vi "ClassAndMethodVIDescriptionEditor.vi"() -> ()   [LabVIEW 2021]
panel:
  in  "Refresh":bool
  in  "Folder Search":string
  in  "Childeren":bool
  in  "Tree":string(tree)
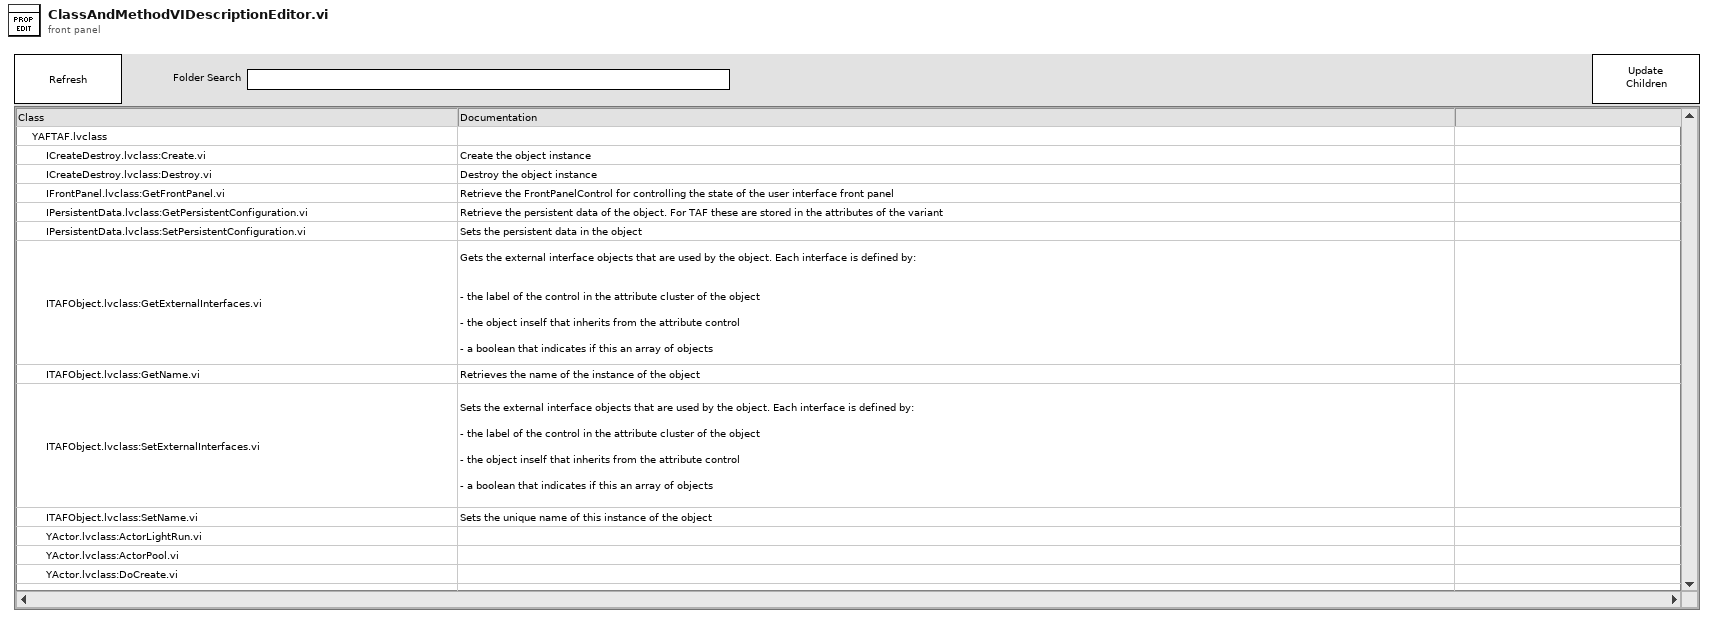
[diagram p1: front panel]
types:
  T1 = enum32{"invalid scope", "public", "private", "protected", "community"}
  T2 = cluster{"Left Cell String":string, "Child Text":string[], "Child Tag":string, "Item Indent":i32, "Child Only?":bool, "Glyph Index":i32}
  T3 = cluster{"Project.ActiveProject":refnum<vi>, "My Computer":refnum<vi>, "All Descendents":refnum<vi>[], "All Descendents":refnum<vi>[], refnum<vi>[]}
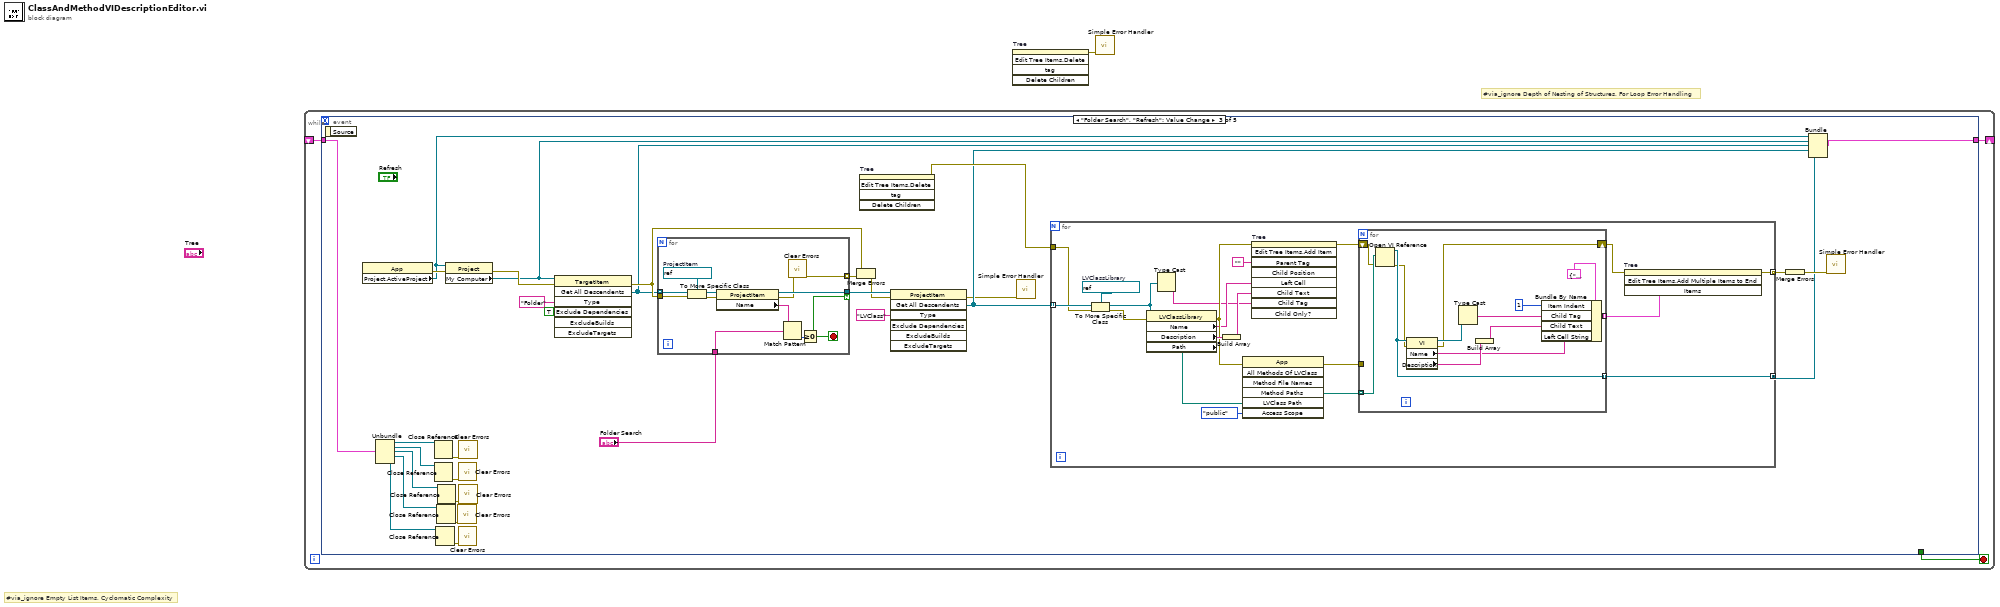
[diagram p0: block diagram]
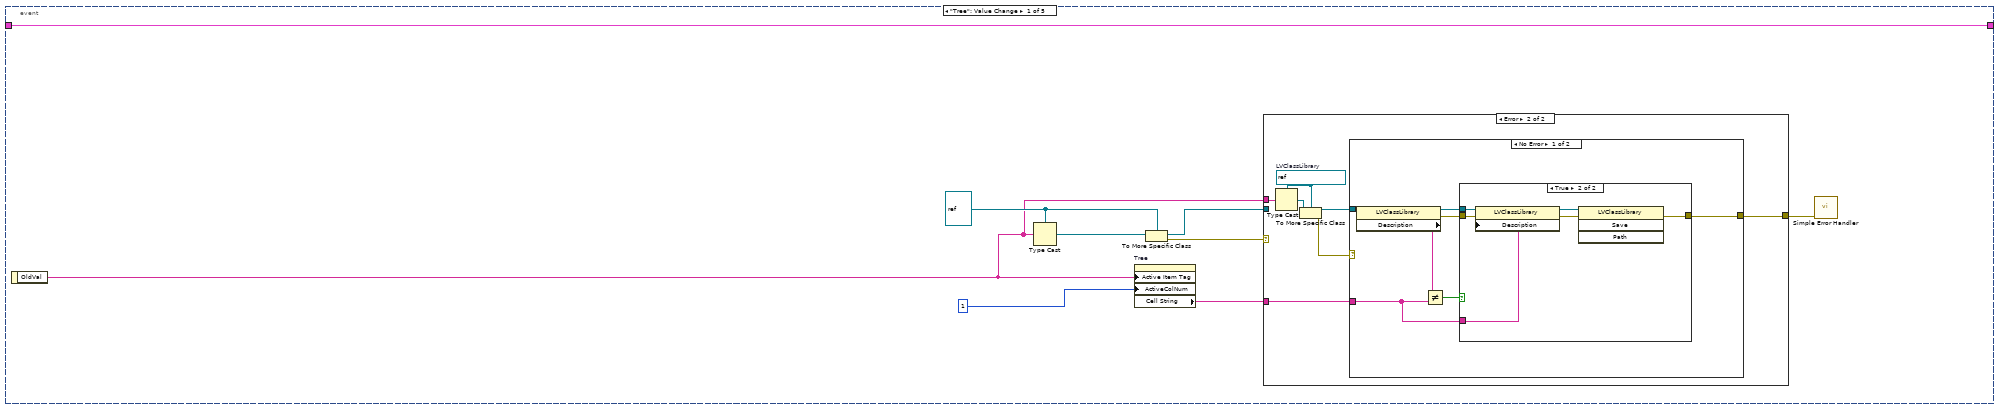
[diagram p2: hidden frame]
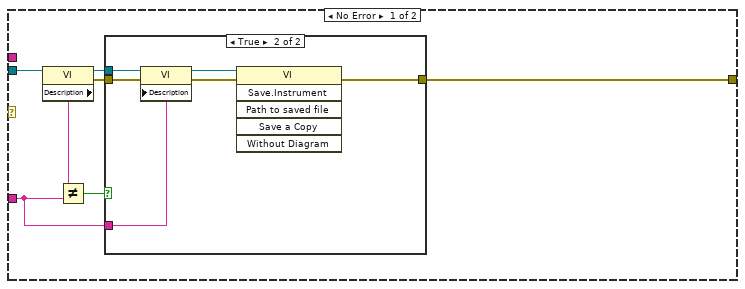
[diagram p3: hidden frame]
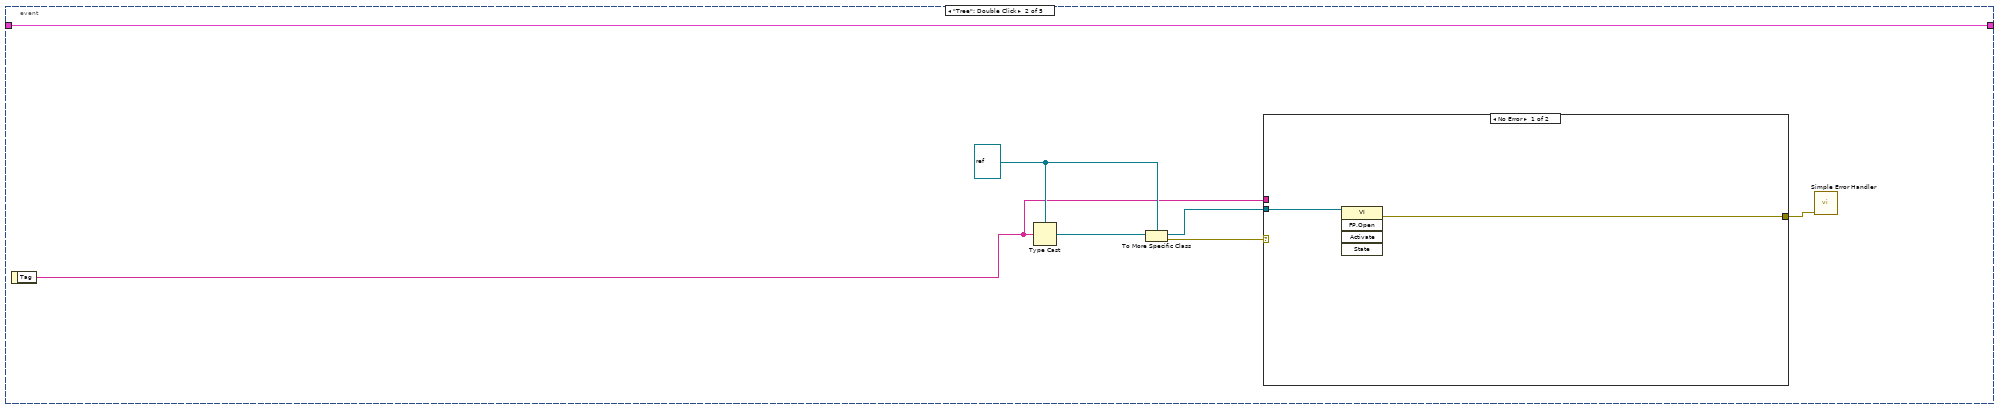
[diagram p7: hidden frame]
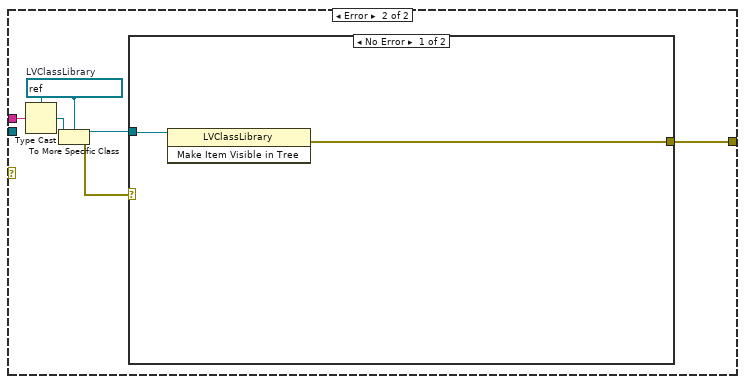
[diagram p8: hidden frame]
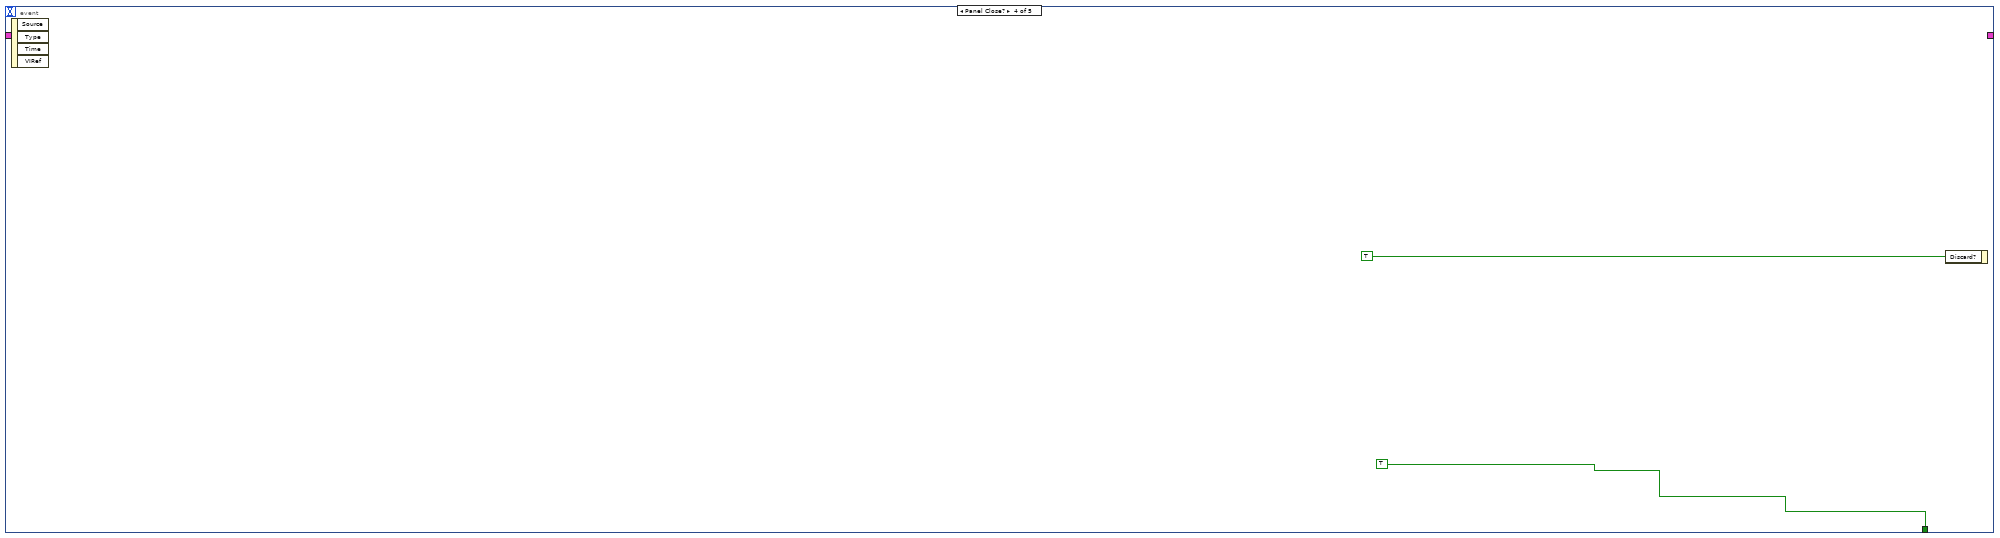
[diagram p10: hidden frame]
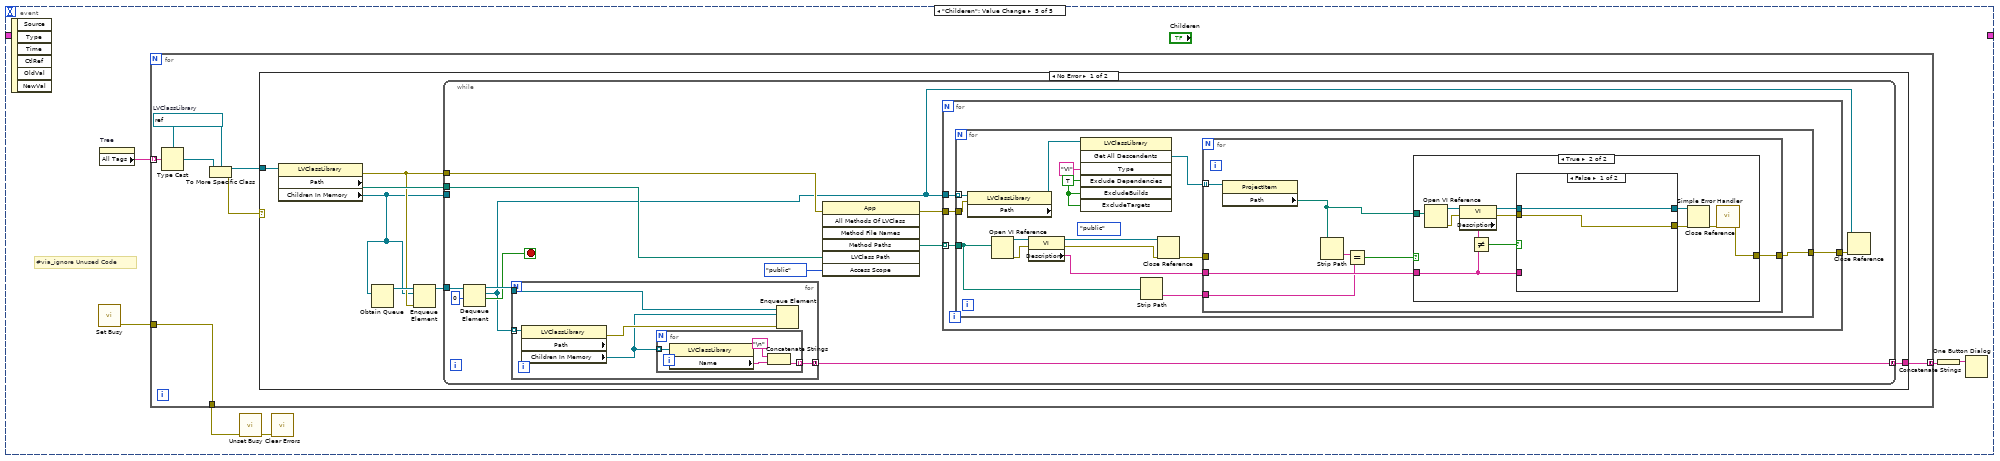
[diagram p11: hidden frame]
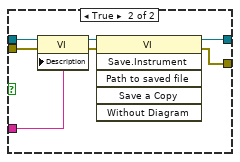
[diagram p13: hidden frame]
diagram:
  # "#via_ignore Depth of Nesting of Structures, For Loop Error Handling"
  # "#via_ignore Empty List Items, Cyclomatic Complexity"
  n1 = while {
    shift-right: [w4] -> _
    shift-left: _ -> [w3]
    stop <- w2 stop-if-true
    n2 = event shown="[2] \"Folder Search\", \"Refresh\": Value Change" {
      selector: _ -> [_ _ _ _ _]
      dyn-events: _ -> [_ _ _ _ _]
      timeout: _ -> [_ _ _ _ _]
      tunnel: [w8 w52 w81 _ _] -> w4
      tunnel: w3 -> [w8 w52 w80 _ _]
      tunnel: [_ _ _ TRUE _] -> w2
      event "Tree": Value Change {
        w12 = refnum<vi> refnum ("reference out")
        n3 = event-data() -> ("OldVal"=w6:string)  [unwired: 1 in]
        n4 = Type Cast(type=w12, x=w6) -> (*(type *) &x=w7:refnum<vi>)
        n5 = property on="Tree" class="Tree (strict)"("Active Item Tag"=w6, "ActiveColNum"=1 ("Active Cell:Active Column Number")) -> ("Cell String"=w9:string)  [unwired: 2 in, 2 out]
        n6 = To More Specific Class(target class=w12, reference=w7) -> (specific class reference=w10:refnum<vi>, error out=w11:errorcluster)  [unwired: 1 in]
        n7 = case shown="Error" w11 {
          tunnel: w10 -> [w20 _]
          tunnel: w9 -> [w16 w34]
          tunnel: w6 -> [_ w31]
          tunnel: [w14 w28] -> w5
          frame No Error {
            n8 = property class="VI"(reference=w20) -> (reference out=w17:refnum<vi>, error out=w15:errorcluster, "Description"=w19:string)  [unwired: 1 in]
            n9 = Not Equal?(x=w19, y=w16) -> (x != y?=w18:bool)
            n10 = case shown="True" w18 {
              tunnel: w17 -> [_ w27]
              tunnel: w16 -> [_ w26]
              tunnel: w15 -> [w21 w23]
              tunnel: [w21 w22] -> w14
              frame False {
              }
              frame True {
                n11 = property class="VI"(reference=w27, error in=w23, "Description"=w26) -> (reference out=w25:refnum<vi>, error out=w24:errorcluster)
                n12 = invoke class="VI" method="Save.Instrument"(reference=w25, error in=w24) -> (error out=w22:errorcluster)  [unwired: 4 in, 5 out]
              }
            }
          }
          frame Error {
            w29 = refnum<vi> refnum  # LVClassLibrary
            n13 = Type Cast(type=w29, x=w31) -> (*(type *) &x=w30:refnum<vi>)
            n14 = To More Specific Class(target class=w29, reference=w30) -> (specific class reference=w33:refnum<vi>, error out=w32:errorcluster)  [unwired: 1 in]
            n15 = case shown="No Error" w32 {
              tunnel: w34 -> [w38 _]
              tunnel: w33 -> [w36 _]
              tunnel: [w35 _] -> w28
              frame No Error {
                n16 = property class="LVClassLibrary"(reference=w36) -> (reference out=w39:refnum<vi>, error out=w37:errorcluster, "Description"=w41:string)  [unwired: 1 in]
                n17 = Not Equal?(x=w41, y=w38) -> (x != y?=w40:bool)
                n18 = case shown="True" w40 {
                  tunnel: w39 -> [_ w48]
                  tunnel: w38 -> [_ w47]
                  tunnel: w37 -> [w42 w44]
                  tunnel: [w42 w43] -> w35
                  frame False {
                  }
                  frame True {
                    n19 = property class="LVClassLibrary"(reference=w48, error in=w44, "Description"=w47) -> (reference out=w46:refnum<vi>, error out=w45:errorcluster)
                    n20 = invoke class="LVClassLibrary" method="Save"(reference=w46, error in=w45) -> (error out=w43:errorcluster)  [unwired: 2 in, 3 out]
                  }
                }
              }
              frame Error {
              }
            }
          }
        }
        n21 = call <vilib>:"Simple Error Handler.vi"("error in (no error)"=w5) -> ()  [unwired: 4 in, 5 out]
      }
      event "Tree": Double Click {
        w55 = refnum<vi> refnum ("reference out")
        n22 = event-data() -> ("Tag"=w50:string)  [unwired: 1 in]
        n23 = Type Cast(type=w55, x=w50) -> (*(type *) &x=w51:refnum<vi>)
        n24 = To More Specific Class(target class=w55, reference=w51) -> (specific class reference=w53:refnum<vi>, error out=w54:errorcluster)  [unwired: 1 in]
        n25 = case shown="No Error" w54 {
          tunnel: w53 -> [w57 _]
          tunnel: w50 -> [_ w61]
          tunnel: [w56 w58] -> w49
          frame No Error {
            n26 = invoke class="VI" method="FP.Open"(reference=w57) -> (error out=w56:errorcluster)  [unwired: 4 in, 4 out]
          }
          frame Error {
            w59 = refnum<vi> refnum  # LVClassLibrary
            n27 = Type Cast(type=w59, x=w61) -> (*(type *) &x=w60:refnum<vi>)
            n28 = To More Specific Class(target class=w59, reference=w60) -> (specific class reference=w63:refnum<vi>, error out=w62:errorcluster)  [unwired: 1 in]
            n29 = case shown="No Error" w62 {
              tunnel: w63 -> [w65 _]
              tunnel: [w64 _] -> w58
              frame No Error {
                n30 = invoke class="LVClassLibrary" method="Make Item Visible in Tree"(reference=w65) -> (error out=w64:errorcluster)  [unwired: 2 in, 2 out]
              }
              frame Error {
              }
            }
          }
        }
        n31 = call <vilib>:"Simple Error Handler.vi"("error in (no error)"=w49) -> ()  [unwired: 4 in, 5 out]
      }
      event "Folder Search", "Refresh": Value Change {
        w88 = TRUE ("ExcludeDependencies")
        n32 = event-data() -> ()  [unwired: 1 in, 1 out]
        n33 = property class="App"() -> (error out=w93:errorcluster, "Project.ActiveProject"=w85:refnum<vi>)  [unwired: 2 in, 1 out]
        n34 = Unbundle(w80) -> ("Project.ActiveProject"=w79:refnum<vi>, "My Computer"=w78:refnum<vi>, "All Descendents"=w77:refnum<vi>[], "All Descendents"=w76:refnum<vi>[], w69:refnum<vi>[])
        n35 = Close Reference(reference=w79) -> (error out=w75:errorcluster)  [unwired: 1 in]
        n36 = Close Reference(reference=w78) -> (error out=w74:errorcluster)  [unwired: 1 in]
        n37 = Close Reference(reference=w69) -> (error out=w71:errorcluster)  [unwired: 1 in]
        n38 = Close Reference(reference=w76) -> (error out=w72:errorcluster)  [unwired: 1 in]
        n39 = Close Reference(reference=w77) -> (error out=w73:errorcluster)  [unwired: 1 in]
        n40 = property class="Project"(reference=w85, error in=w93) -> (error out=w94:errorcluster, "My Computer"=w84:refnum<vi>)  [unwired: 1 out]
        n41 = call <vilib>:"Clear Errors.vi"("error in (no error)"=w72) -> ()  [unwired: 5 in, 2 out]
        n42 = call <vilib>:"Clear Errors.vi"("error in (no error)"=w74) -> ()  [unwired: 5 in, 2 out]
        n43 = call <vilib>:"Clear Errors.vi"("error in (no error)"=w71) -> ()  [unwired: 5 in, 2 out]
        n44 = call <vilib>:"Clear Errors.vi"("error in (no error)"=w75) -> ()  [unwired: 5 in, 2 out]
        n45 = call <vilib>:"Clear Errors.vi"("error in (no error)"=w73) -> ()  [unwired: 5 in, 2 out]
        n46 = invoke class="TargetItem" method="Get All Descendents"(reference=w84, error in=w94, "Type"="Folder", "Exclude Dependencies"=w88, "ExcludeBuilds"=w88, "ExcludeTargets"=w88) -> (error out=w95:errorcluster, "All Descendents"=w83:refnum<vi>[])  [unwired: 1 in, 5 out]
        n47 = for {
          tunnel: w83 -> [w141] mode=indexing
          tunnel: [w136] -> w91 if=w134
          tunnel: w95 -> [w133]
          tunnel: "Folder Search" -> [w131]
          tunnel: [w130] -> w66 mode=indexing
          stop <- w134 stop-if-true
          w140 = refnum<vi> refnum  # ProjectItem
          n48 = To More Specific Class(target class=w140, reference=w141, error in=w133) -> (specific class reference=w139:refnum<vi>, error out=w138:errorcluster)
          n49 = property class="ProjectItem"(reference=w139, error in=w138) -> (reference out=w136:refnum<vi>, error out=w132:errorcluster, "Name"=w137:string)
          n50 = Match Pattern(string=w137, regular expression=w131) -> (offset past match=w135:i32)  [unwired: 1 in, 3 out]
          n51 = call <vilib>:"Clear Errors.vi"("error in (no error)"=w132) -> ("error out"=w130:errorcluster)  [unwired: 5 in, 1 out]
          n52 = Greater Or Equal To 0?(x=w135) -> (x >= 0?=w134:bool)
        }
        n53 = Merge Errors(w95, w66) -> (w67:errorcluster)
        n54 = invoke on="Tree" class="Tree (strict)" method="Edit Tree Items.Delete"() -> (error out=w92:errorcluster)  [unwired: 5 in, 4 out]
        n55 = invoke class="ProjectItem" method="Get All Descendents"(reference=w91, error in=w67, "Type"="LVClass") -> (error out=w68:errorcluster, "All Descendents"=w82:refnum<vi>[])  [unwired: 4 in, 5 out]
        n56 = call <vilib>:"Simple Error Handler.vi"("error in (no error)"=w68) -> ()  [unwired: 4 in, 5 out]
        n57 = for {
          tunnel: w82 -> [w116] mode=indexing
          tunnel: w92 -> [w101]
          tunnel: [w108] -> w87 mode=indexing
          tunnel: [w104] -> w70 mode=concatenating
          w115 = refnum<vi> refnum  # LVClassLibrary
          n58 = To More Specific Class(target class=w115, reference=w116, error in=w101) -> (specific class reference=w112:refnum<vi>, error out=w111:errorcluster)
          n59 = property class="LVClassLibrary"(reference=w112, error in=w111) -> (error out=w103:errorcluster, "Name"=w98:string, "Description"=w113:string, "Path"=w107:path)  [unwired: 1 out]
          n60 = Type Cast(x=w112) -> (*(type *) &x=w97:string)  [unwired: 1 in]
          n61 = Build Array(w113) -> (w100:string[])
          n62 = invoke class="App" method="All Methods Of LVClass"(error in=w103, "LVClass Path"=w107, "Access Scope"=T1."public") -> (error out=w102:errorcluster, "Method Paths"=w105:path[])  [unwired: 4 in, 5 out]
          n63 = invoke on="Tree" class="Tree (strict)" method="Edit Tree Items.Add Item"(error in=w103, "Parent Tag"="", "Left Cell"=w98, "Child Text"=w100, "Child Tag"=w97) -> (error out=w110:errorcluster)  [unwired: 4 in, 8 out]
          n64 = for {
            tunnel: [w127] -> w114 mode=indexing
            shift-right: [w121] -> w109
            shift-left: w110 -> [w118]
            tunnel: w105 -> [w120] mode=indexing
            tunnel: [w119] -> w104 mode=indexing
            tunnel: w102 -> [_]
            n65 = Open VI Reference(vi path=w120, error in (no error)=w118) -> (vi reference=w119:refnum<vi>, error out=w117:errorcluster)  [unwired: 4 in]
            n66 = property class="VI"(reference=w119, error in=w117) -> (reference out=w122:refnum<vi>, error out=w121:errorcluster, "Name"=w124:string, "Description"=w126:string)
            n67 = Type Cast(x=w122) -> (*(type *) &x=w123:string)  [unwired: 1 in]
            n68 = Build Array(w126) -> (w125:string[])
            n69 = Bundle By Name(cluster=T2 {"Left Cell String"="", "Child Text"=[], "Child Tag"="", "Item Indent"=0, "Child Only?"=FALSE, "Glyph Index"=0} ("Item"), "Item Indent"=1, "Child Tag"=w123, "Child Text"=w125, "Left Cell String"=w124) -> (w127:T2)
          }
          n70 = invoke on="Tree" class="Tree (strict)" method="Edit Tree Items.Add Multiple Items to End"(error in=w109, "Items"=w114) -> (error out=w108:errorcluster)  [unwired: 2 in, 3 out]
        }
        n71 = Merge Errors(w87) -> (w86:errorcluster)
        n72 = Bundle("Project.ActiveProject"=w85, "My Computer"=w84, "All Descendents"=w83, "All Descendents"=w82, w70) -> (w81:T3)  [unwired: 1 in]
        n73 = call <vilib>:"Simple Error Handler.vi"("error in (no error)"=w86) -> ()  [unwired: 4 in, 5 out]
      }
      event Panel Close? {
        n74 = event-data() -> ()  [unwired: 1 in, 4 out]
        n75 = event-data("Discard?"=TRUE) -> ()  [unwired: 1 in, 1 out]
      }
      event "Childeren": Value Change {
        # "#via_ignore Unused Code"
        n76 = event-data() -> ()  [unwired: 1 in, 6 out]
        n77 = call <vilib>:"Set Busy.vi"() -> ("error out"=w148:errorcluster)  [unwired: 10 in, 1 out]
        n78 = property on="Tree" class="Tree (strict)"() -> ("All Tags"=w149:string[])  [unwired: 2 in, 2 out]
        n79 = for {
          tunnel: w149 -> [w152] mode=indexing
          tunnel: [w151] -> w147
          tunnel: w148 -> [w151]
          tunnel: [w150] -> w145 mode=concatenating
          w153 = refnum<vi> refnum  # LVClassLibrary
          n80 = Type Cast(type=w153, x=w152) -> (*(type *) &x=w156:refnum<vi>)
          n81 = To More Specific Class(target class=w153, reference=w156) -> (specific class reference=w154:refnum<vi>, error out=w155:errorcluster)  [unwired: 1 in]
          n82 = case shown="No Error" w155 {
            tunnel: w154 -> [w163 _]
            tunnel: [w157 _] -> w150
            frame No Error {
              n83 = property class="LVClassLibrary"(reference=w163) -> (error out=w159:errorcluster, "Path"=w160:path, "Children In Memory"=w158:refnum<vi>[])  [unwired: 1 in, 1 out]
              n84 = Obtain Queue(element data type=w158) -> (queue out=w162:refnum<queue>)  [unwired: 4 in, 2 out]
              n85 = Enqueue Element(queue=w162, element=w158, error in (no error)=w159) -> (queue out=w161:refnum<queue>)  [unwired: 1 in, 2 out]
              n86 = while {
                tunnel: w160 -> [w166]
                tunnel: w159 -> [w173]
                tunnel: w158 -> [_]
                tunnel: w161 -> [w170]
                tunnel: [w164] -> w157 mode=concatenating
                stop <- w168 stop-if-true
                n87 = Dequeue Element(queue=w170, timeout in ms (-1)=0) -> (queue out=w169:refnum<queue>, element=w165:refnum<vi>[], timed out?=w168:bool)  [unwired: 1 in, 1 out]
                n88 = for {
                  tunnel: w165 -> [w180] mode=indexing
                  tunnel: w169 -> [w179]
                  tunnel: [w176] -> w164 mode=concatenating
                  n89 = property class="LVClassLibrary" props=["Path", "Children In Memory"](reference=w180) -> (error out=w178:errorcluster, "Children In Memory"=w177:refnum<vi>[])  [unwired: 1 in, 2 out]
                  n90 = for {
                    tunnel: w177 -> [w184] mode=indexing
                    tunnel: [w182] -> w176 mode=indexing
                    n91 = property class="LVClassLibrary"(reference=w184) -> ("Name"=w183:string)  [unwired: 1 in, 2 out]
                    n92 = Concatenate Strings("\n", w183) -> (w182:string)
                  }
                  n93 = Enqueue Element(queue=w179, element=w177, error in (no error)=w178) -> ()  [unwired: 1 in, 3 out]
                }
                n94 = invoke class="App" method="All Methods Of LVClass"(error in=w173, "LVClass Path"=w166, "Access Scope"=T1."public") -> (error out=w172:errorcluster, "Method Paths"=w174:path[])  [unwired: 4 in, 5 out]
                n95 = for {
                  tunnel: w174 -> [w187] mode=indexing
                  tunnel: w165 -> [w188]
                  tunnel: w172 -> [w186]
                  tunnel: [w185] -> w171
                  n96 = for {
                    tunnel: w188 -> [w201] mode=indexing
                    tunnel: w187 -> [w197]
                    tunnel: w186 -> [w195]
                    tunnel: [w194] -> w185
                    w189 = TRUE ("ExcludeDependencies")
                    (unwired) T1."public" ("Access Scope")
                    n97 = property class="LVClassLibrary" props=["Path"](reference=w201, error in=w195) -> (reference out=w192:refnum<vi>)  [unwired: 2 out]
                    n98 = Open VI Reference(vi path=w197) -> (vi reference=w203:refnum<vi>, error out=w202:errorcluster)  [unwired: 5 in]
                    n99 = property class="VI"(reference=w203, error in=w202) -> (reference out=w199:refnum<vi>, error out=w200:errorcluster, "Description"=w198:string)
                    n100 = invoke class="LVClassLibrary" method="Get All Descendents"(reference=w192, "Type"="VI", "Exclude Dependencies"=w189, "ExcludeBuilds"=w189, "ExcludeTargets"=w189) -> ("All Descendents"=w190:refnum<vi>[])  [unwired: 2 in, 6 out]
                    n101 = Strip Path(path=w197) -> (name=w196:string)  [unwired: 1 out]
                    n102 = Close Reference(reference=w199, error in (no error)=w200) -> (error out=w193:errorcluster)
                    n103 = for {
                      tunnel: w198 -> [w210]
                      tunnel: w196 -> [w207]
                      tunnel: [w206] -> w194
                      tunnel: w190 -> [w205] mode=indexing
                      tunnel: w193 -> [_]
                      n104 = property class="ProjectItem"(reference=w205) -> ("Path"=w204:path)  [unwired: 1 in, 2 out]
                      n105 = Strip Path(path=w204) -> (name=w208:string)  [unwired: 1 out]
                      n106 = Equal?(x=w208, y=w207) -> (x = y?=w209:bool)
                      n107 = case shown="True" w209 {
                        tunnel: w210 -> [_ w213]
                        tunnel: w204 -> [_ w222]
                        tunnel: [_ w211] -> w206
                        frame False {
                        }
                        frame True {
                          n108 = Open VI Reference(vi path=w222) -> (vi reference=w218:refnum<vi>, error out=w217:errorcluster)  [unwired: 5 in]
                          n109 = property class="VI"(reference=w218, error in=w217) -> (reference out=w215:refnum<vi>, error out=w216:errorcluster, "Description"=w214:string)
                          n110 = Not Equal?(x=w214, y=w213) -> (x != y?=w212:bool)
                          n111 = case shown="False" w212 {
                            tunnel: w213 -> [_ w231]
                            tunnel: [w224 w228] -> w221
                            tunnel: [w223 w227] -> w220
                            tunnel: w216 -> [w223 w226]
                            tunnel: w215 -> [w224 w225]
                            frame False {
                            }
                            frame True {
                              n112 = property class="VI"(reference=w225, error in=w226, "Description"=w231) -> (reference out=w230:refnum<vi>, error out=w229:errorcluster)
                              n113 = invoke class="VI" method="Save.Instrument"(reference=w230, error in=w229) -> (reference out=w228:refnum<vi>, error out=w227:errorcluster)  [unwired: 4 in, 4 out]
                            }
                          }
                          n114 = Close Reference(reference=w221, error in (no error)=w220) -> (error out=w219:errorcluster)
                          n115 = call <vilib>:"Simple Error Handler.vi"("error in (no error)"=w219) -> ("error out"=w211:errorcluster)  [unwired: 4 in, 4 out]
                        }
                      }
                    }
                  }
                }
                n116 = Close Reference(reference=w165, error in (no error)=w171) -> ()  [unwired: 1 out]
              }
            }
            frame Error {
            }
          }
        }
        n117 = call <vilib>:"Unset Busy.vi"("error in (no error)"=w147) -> ("error out"=w146:errorcluster)  [unwired: 10 in]
        n118 = call <vilib>:"Clear Errors.vi"("error in (no error)"=w146) -> ()  [unwired: 5 in, 2 out]
        n119 = Concatenate Strings(w145) -> (w144:string)
        n120 = One Button Dialog(message=w144) -> ()  [unwired: 1 in, 1 out]
      }
    }
  }
  n121 = invoke on="Tree" class="Tree (strict)" method="Edit Tree Items.Delete"() -> (error out=w1:errorcluster)  [unwired: 5 in, 4 out]
  n122 = call <vilib>:"Simple Error Handler.vi"("error in (no error)"=w1) -> ()  [unwired: 4 in, 5 out]
